vi "peirce_main.vi"(7 "StressDist_types":T1, 8 "Error In":errorcluster, 11 "main_FGV_data":T2={"pipe_properties"={"out_radius"=0.0, "in_radius"=0.0, "out_diameter"=0.0, "in_diameter"=0.0, "thickness"=0.0, "inertia"=0.0, "area"=0.0}, "DirPath"=path "L:/Documentos/00 SERVIÇOS/Tensão residual/Olapa 10-2017/Dados/Primeira Seção/Furos", "DirReport"=path "L:/Documentos/00 SERVIÇOS/Tensão residual/Olapa 10-2017/RelatóriosOlapa/Teste", "Points"=[], "ovalization_data"={"AngOval"=[0.0, 60.0, 120.0, 22.5, 45.0, 67.5, 90.0, 112.5, 135.0, 157.5, 180.0], "OvalDiam"=[324.25, 324.6, 324.55, 324.25, 324.55, 324.65, 324.6, 324.65, 324.55, 324.5, 324.4], "Plots"={"Ref"={"X"=[], "Y"=[]}, "Elipse"={"X"=[], "Y"=[]}, "Points"={"X"=[], "Y"=[]}}, "Ampliation"=100.0, "Results"={"MD"=0.0, "mD"=0.0, "Dmed"=0.0, "Oval"=0.0, "ang"=0.0, "X0"=0.0, "Y0"=0.0}}, "StressDist_data"={"Long"={"Plot"=[], "Fit"=[], "ColorMap"=[], "Data"=[], "peirce_data"={"Plot"=[], "Index removidos"=[]}}, "Circ"={"Plot"=[], "Fit"=[], "ColorMap"=[], "Data"=[], "peirce_data"={"Plot"=[], "Index removidos"=[]}}, "Shear"={"Plot"=[], "Fit"=[], "ColorMap"=[], "Data"=[], "peirce_data"={"Plot"=[], "Index removidos"=[]}}, "Equivalent"={"Plot"=[], "Fit"=[], "ColorMap"=[], "Data"=[], "peirce_data"={"Plot"=[], "Index removidos"=[]}}}, "pressure_data"={"Pressure"=[], "StressCircOval"=[], "StressCirc"=[], "StressLong"=[], "Plot"=[], "Angle"=[]}}) -> (0 "Error Out":errorcluster, 3 "main_FGV_data-out":T2={"pipe_properties"={"out_radius"=0.0, "in_radius"=0.0, "out_diameter"=0.0, "in_diameter"=0.0, "thickness"=0.0, "inertia"=0.0, "area"=0.0}, "DirPath"=path "L:/Documentos/00 SERVIÇOS/Tensão residual/Olapa 10-2017/Dados/Primeira Seção/Furos", "DirReport"=path "L:/Documentos/00 SERVIÇOS/Tensão residual/Olapa 10-2017/RelatóriosOlapa/Teste", "Points"=[], "ovalization_data"={"AngOval"=[0.0, 60.0, 120.0, 22.5, 45.0, 67.5, 90.0, 112.5, 135.0, 157.5, 180.0], "OvalDiam"=[324.25, 324.6, 324.55, 324.25, 324.55, 324.65, 324.6, 324.65, 324.55, 324.5, 324.4], "Plots"={"Ref"={"X"=[], "Y"=[]}, "Elipse"={"X"=[], "Y"=[]}, "Points"={"X"=[], "Y"=[]}}, "Ampliation"=100.0, "Results"={"MD"=0.0, "mD"=0.0, "Dmed"=0.0, "Oval"=0.0, "ang"=0.0, "X0"=0.0, "Y0"=0.0}}, "StressDist_data"={"Long"={"Plot"=[], "Fit"=[], "ColorMap"=[], "Data"=[], "peirce_data"={"Plot"=[], "Index removidos"=[]}}, "Circ"={"Plot"=[], "Fit"=[], "ColorMap"=[], "Data"=[], "peirce_data"={"Plot"=[], "Index removidos"=[]}}, "Shear"={"Plot"=[], "Fit"=[], "ColorMap"=[], "Data"=[], "peirce_data"={"Plot"=[], "Index removidos"=[]}}, "Equivalent"={"Plot"=[], "Fit"=[], "ColorMap"=[], "Data"=[], "peirce_data"={"Plot"=[], "Index removidos"=[]}}}, "pressure_data"={"Pressure"=[], "StressCircOval"=[], "StressCirc"=[], "StressLong"=[], "Plot"=[], "Angle"=[]}})   [LabVIEW 2016]
uses:
  MainFGV/main_FGV_data.ctl
  MainFGV/pipe_properties.ctl
  StressCalculations/point_data.ctl
  Ovalization/ovalization_data.ctl
  StressDist_data.ctl
  StressDist_single_data.ctl
  peirce_data.ctl
  Pressure/pressure_data.ctl
  StressDist_types.ctl
  Report/report_mods.ctl
panel:
  out "Desvios":cluster{dbl[], dbl[]}[](graph) caption="Ovalização"
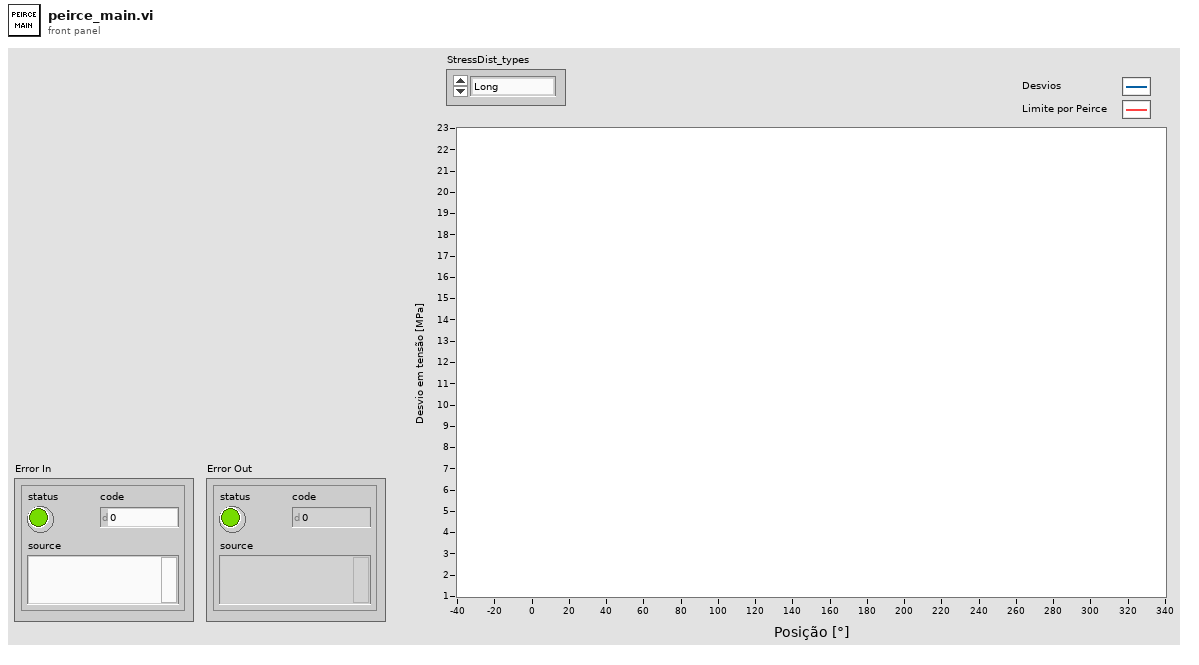
[diagram p1: front panel]
types:
  T1 = typedef "StressDist_types.ctl" = enum16{"Long", "Circ", "Shear", "Equivalent"}
  T2 = typedef "main_FGV_data.ctl" = cluster{"pipe_properties":T3, "DirPath":path, "DirReport":path, "Points":T4[], "ovalization_data":T5, "StressDist_data":T6, "pressure_data":T9}
  T3 = typedef "pipe_properties.ctl" = cluster{"out_radius":dbl, "in_radius":dbl, "out_diameter":dbl, "in_diameter":dbl, "thickness":dbl, "inertia":dbl, "area":dbl}
  T4 = typedef "point_data.ctl" = cluster{"LongStress":dbl, "CircStress":dbl, "ShearStress":dbl, "Pressure":dbl, "Angle":dbl, "Thickness":dbl, "HoleDiam":dbl, "EquiStress":dbl, "S1":dbl, "S2":dbl, "Beta":dbl}
  T5 = typedef "ovalization_data.ctl" = cluster{"AngOval":dbl[], "OvalDiam":dbl[], "Plots":cluster{"Ref":cluster{"X":dbl[], "Y":dbl[]}, "Elipse":cluster{"X":dbl[], "Y":dbl[]}, "Points":cluster{"X":dbl[], "Y":dbl[]}}, "Ampliation":dbl, "Results":cluster{"MD":dbl, "mD":dbl, "Dmed":dbl, "Oval":dbl, "ang":dbl, "X0":dbl, "Y0":dbl}}
  T6 = typedef "StressDist_data.ctl" = cluster{"Long":T7, "Circ":T7, "Shear":T7, "Equivalent":T7}
  T7 = typedef "StressDist_single_data.ctl" = cluster{"Plot":cluster{"Angle":dbl[], "Stress":dbl[]}[], "Fit":dbl[], "ColorMap":dbl[][], "Data":string[][], "peirce_data":T8}
  T8 = typedef "peirce_data.ctl" = cluster{"Plot":cluster{"Array":dbl[], "Array":dbl[]}[], "Index removidos":i32[]}
  T9 = typedef "pressure_data.ctl" = cluster{"Pressure":dbl[], "StressCircOval":dbl[], "StressCirc":dbl[], "StressLong":dbl[], "Plot":cluster{"Angle":dbl[], "Stress":dbl[]}[], "Angle":dbl[]}
  T10 = typedef "report_mods.ctl" = enum16{"Init", "Table", "Graph", "TablefromGraph", "End"}
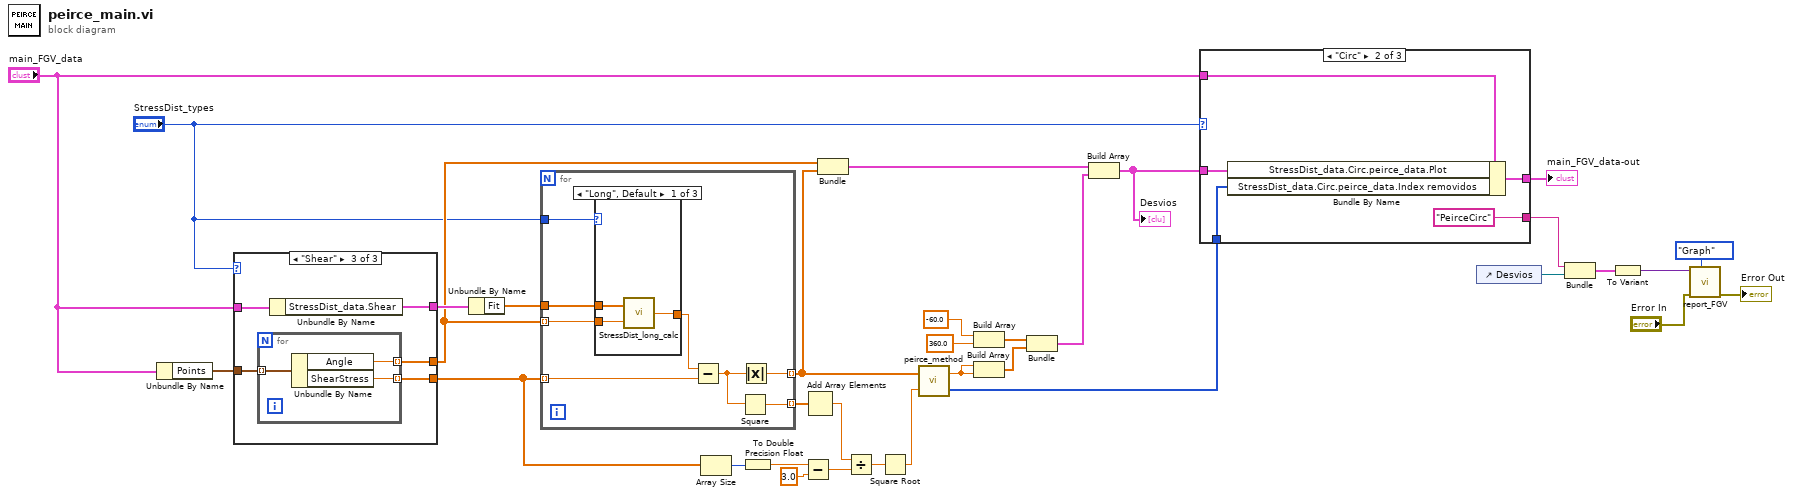
[diagram p0: block diagram]
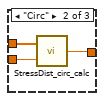
[diagram p2: hidden frame]
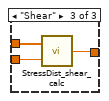
[diagram p3: hidden frame]
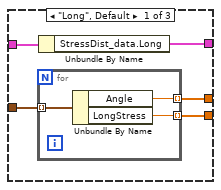
[diagram p4: hidden frame]
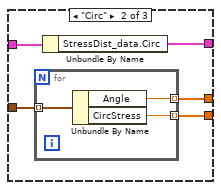
[diagram p5: hidden frame]
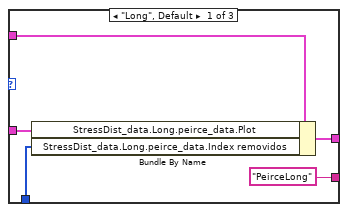
[diagram p6: hidden frame]
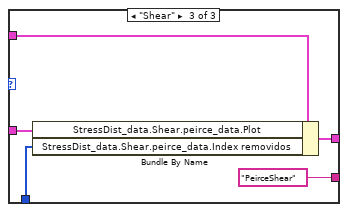
[diagram p7: hidden frame]
diagram:
  n1 = Unbundle By Name("main_FGV_data") -> ("Points"=w32:T4[])
  n2 = case shown="\"Shear\"" "StressDist_types" {
    tunnel: "main_FGV_data" -> [w38 w46 w54]
    tunnel: [w37 w45 w53] -> w33
    tunnel: w32 -> [w36 w44 w52]
    tunnel: [w35 w43 w51] -> w23
    tunnel: [w34 w42 w50] -> w25
    frame "Long", Default {
      n3 = for {
        tunnel: w36 -> [w41] mode=indexing
        tunnel: [w40] -> w35 mode=indexing
        tunnel: [w39] -> w34 mode=indexing
        n4 = Unbundle By Name(w41) -> ("Angle"=w40:dbl, "LongStress"=w39:dbl)
      }
      n5 = Unbundle By Name(w38) -> ("StressDist_data.Long"=w37:T7)
    }
    frame "Circ" {
      n6 = for {
        tunnel: w44 -> [w49] mode=indexing
        tunnel: [w48] -> w43 mode=indexing
        tunnel: [w47] -> w42 mode=indexing
        n7 = Unbundle By Name(w49) -> ("Angle"=w48:dbl, "CircStress"=w47:dbl)
      }
      n8 = Unbundle By Name(w46) -> ("StressDist_data.Circ"=w45:T7)
    }
    frame "Shear" {
      n9 = for {
        tunnel: w52 -> [w57] mode=indexing
        tunnel: [w56] -> w51 mode=indexing
        tunnel: [w55] -> w50 mode=indexing
        n10 = Unbundle By Name(w57) -> ("Angle"=w56:dbl, "ShearStress"=w55:dbl)
      }
      n11 = Unbundle By Name(w54) -> ("StressDist_data.Shear"=w53:T7)
    }
  }
  n12 = Unbundle By Name(w33) -> ("Fit"=w31:dbl[])
  n13 = for {
    tunnel: w31 -> [w64]
    tunnel: "StressDist_types" -> [w65]
    tunnel: w23 -> [w63] mode=indexing
    tunnel: w25 -> [w61] mode=indexing
    tunnel: [w59] -> w22 mode=indexing
    tunnel: [w58] -> w24 mode=indexing
    n14 = case shown="\"Long\", Default" w65 {
      tunnel: w64 -> [w67 w71 w74]
      tunnel: w63 -> [w68 w70 w73]
      tunnel: [w66 w69 w72] -> w62
      frame "Long", Default {
        n15 = call "StressDist_long_calc.vi"("Angle"=w68, "Parameters"=w67) -> ("Stress"=w66:dbl)
      }
      frame "Circ" {
        n16 = call "StressDist_circ_calc.vi"("Angle"=w70, "Parameters"=w71) -> ("Stress"=w69:dbl)
      }
      frame "Shear" {
        n17 = call "StressDist_shear_calc.vi"("Angle"=w73, "Parameters"=w74) -> ("Stress"=w72:dbl)
      }
    }
    n18 = Subtract(x=w62, y=w61) -> (x-y=w60:dbl)
    n19 = Square(x=w60) -> (x^2=w58:dbl)
    n20 = Absolute Value(x=w60) -> (abs(x)=w59:dbl)
  }
  n21 = Array Size(array=w25) -> (size(s)=w30:i32)
  n22 = To Double Precision Float(number=w30) -> (double precision float=w26:dbl)
  n23 = Subtract(x=w26, y=3.0) -> (x-y=w28:dbl)
  n24 = Add Array Elements(numeric array=w24) -> (sum=w15:dbl)
  n25 = Bundle(w23, w22) -> (w17:cluster{dbl[], dbl[]})  [unwired: 1 in]
  n26 = Divide(x=w15, y=w28) -> (x/y=w29:dbl)
  n27 = Square Root(x=w29) -> (sqrt(x)=w14:dbl)
  n28 = call "peirce_method.vi"("DesvioPadrão"=w14, "DesviosAbsolutos"=w22) -> ("IndexRemovidos"=w9:i32[], "PeirceTol"=w21:dbl)
  n29 = Build Array(-60.0 ("element"), 360.0 ("element")) -> (w19:dbl[])
  n30 = Build Array(w21, w21) -> (w18:dbl[])
  n31 = Bundle(w19, w18) -> (w16:cluster{dbl[], dbl[]})  [unwired: 1 in]
  n32 = Build Array(w17, w16) -> (w10:cluster{dbl[], dbl[]}[])
  "Desvios" <- w10
  n33 = case shown="\"Circ\"" "StressDist_types" {
    tunnel: "main_FGV_data" -> [w79 w83 w88]
    tunnel: w10 -> [w78 w82 w87]
    tunnel: w9 -> [w77 w81 w86]
    tunnel: [w76 w84 w89] -> w8
    tunnel: ["PeirceLong" "PeirceCirc" "PeirceShear"] -> w3
    frame "Long", Default {
      n34 = Bundle By Name(cluster=w79, "StressDist_data.Long.peirce_data.Plot"=w78, "StressDist_data.Long.peirce_data.Index removidos"=w77) -> (w76:T2)
    }
    frame "Circ" {
      n35 = Bundle By Name(cluster=w83, "StressDist_data.Circ.peirce_data.Plot"=w82, "StressDist_data.Circ.peirce_data.Index removidos"=w81) -> (w84:T2)
    }
    frame "Shear" {
      n36 = Bundle By Name(cluster=w88, "StressDist_data.Shear.peirce_data.Plot"=w87, "StressDist_data.Shear.peirce_data.Index removidos"=w86) -> (w89:T2)
    }
  }
  "main_FGV_data-out" <- w8
  n37 = control-ref of="Desvios"() -> (w4:refnum<vi>)
  n38 = Bundle(w3, "Desvios"=w4) -> (w6:cluster{string, "Desvios":refnum<vi>})  [unwired: 1 in]
  n39 = To Variant(anything=w6) -> (Variant=w5:variant)
  n40 = call "report_FGV.vi"("report_mods"=report_mods."Graph", "Error In"="Error In", "Data in"=w5) -> ("Error Out"=→"Error Out":errorcluster)  [unwired: 8 in]
